vi "Function Generator.vi"() -> ()   [LabVIEW 2024]
uses:
  <vilib>/Instr/_visa.llb/VISA Configure Serial Port (Instr).vi
  <vilib>/measure/NI_MABase.lvlib
panel:
  in  "Tab Control":enum32{"Page 1", "Page 2"}(tab)
  in  "VISA resource name":refnum<visa-resource-name>
  in  "frequency * 100":dbl(knob) scale=0.0..20.0
  in  "signal type":T1(ring)
  in  "stop":bool
  out "Waveform Chart":waveform(dbl)(graph)
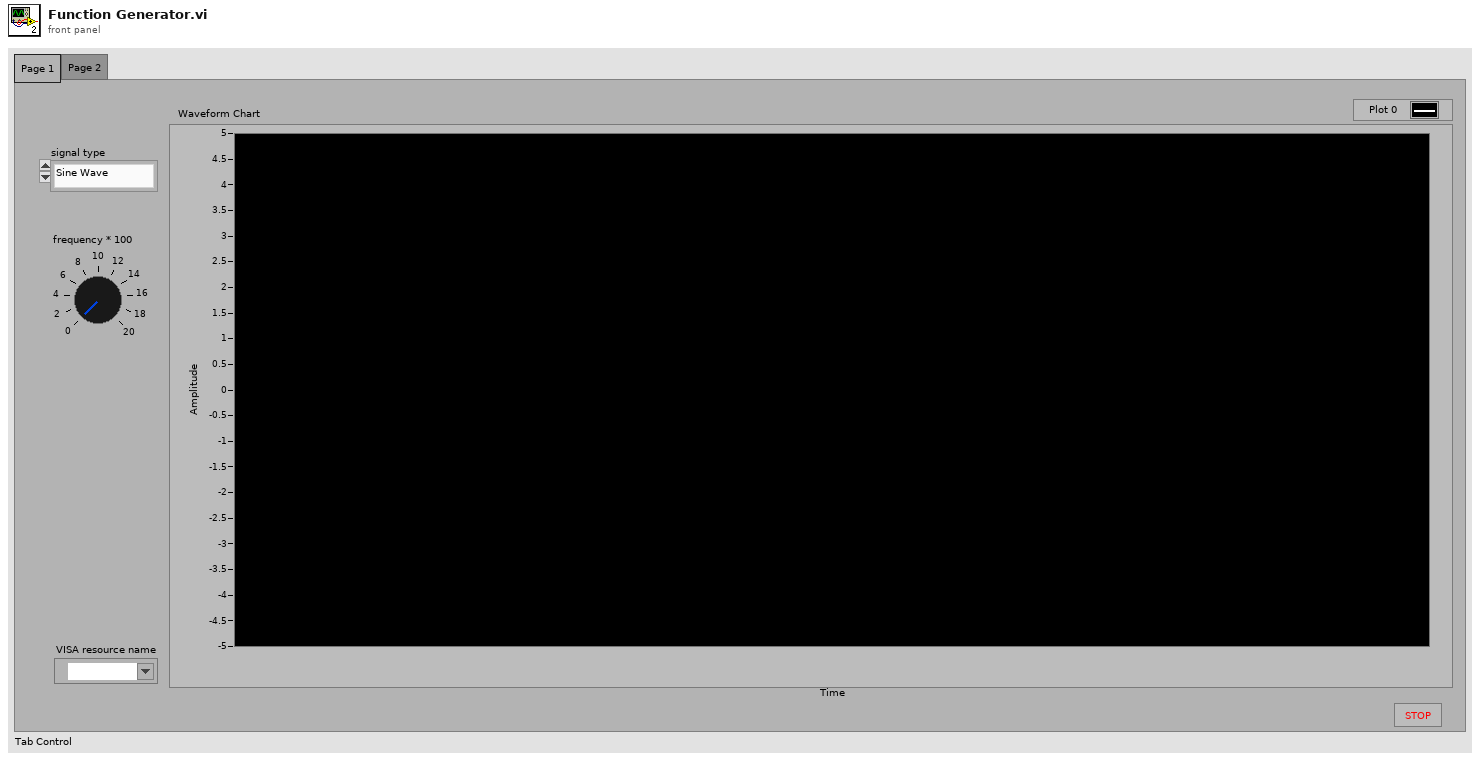
[diagram p1: front panel]
types:
  T1 = enum16{"Sine Wave", "Triangle Wave", "Square Wave", "Sawtooth Wave"}
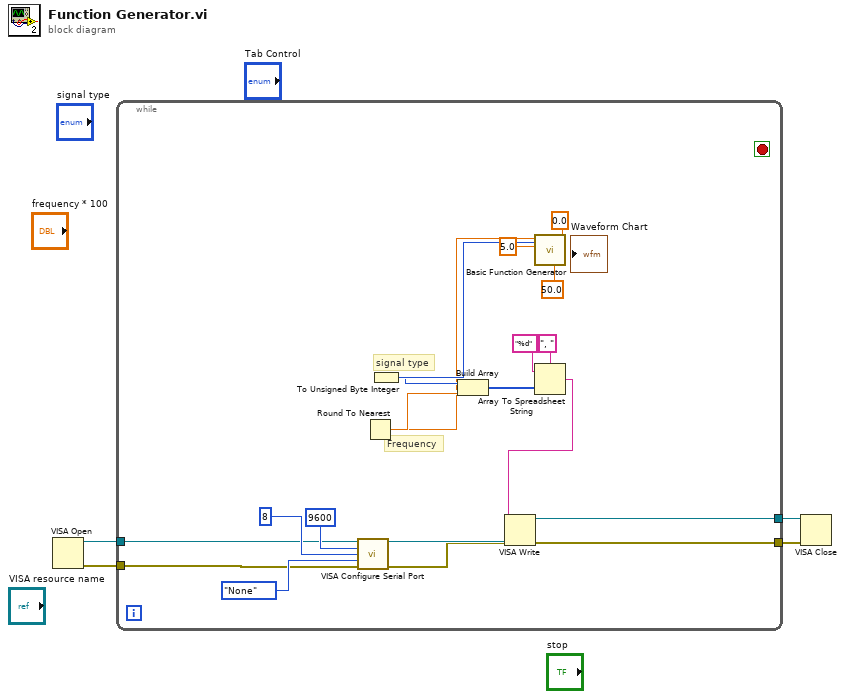
[diagram p0: block diagram]
diagram:
  n1 = VISA Open() -> (VISA resource name=w2:refnum<visa-resource-name>, error out=w1:errorcluster)  [unwired: 5 in]
  n2 = while {
    tunnel: [w24] -> w4
    tunnel: [w23] -> w3
    tunnel: w2 -> [w6]
    tunnel: w1 -> [w5]
    stop <- _ stop-if-true
    # "Frequency"
    # "signal type"
    n3 = call-poly "VISA Configure Serial Port"("VISA resource name"=w6, "baud rate (9600)"=u32 9600, "data bits (8)"=u16 8, "parity (0:none)"=enum16{"None", "Odd", "Even", "Mark", "Space"}."None", "error in (no error)"=w5) -> ("VISA resource name out"=w12:refnum<visa-resource-name>, "error out"=w11:errorcluster)  [unwired: 9 in]
    n4 = call <vilib>:"Basic Function Generator.vi"("offset"=0.0, "square wave duty cycle (%)"=50.0, "amplitude"=5.0) -> ("signal out"=w25:waveform(dbl), "signal type"=w22:T1, "frequency"=w7:dbl)  [unwired: 4 in, 2 out]
    n5 = Round To Nearest(number=w7) -> (nearest integer value=w20:dbl)
    n6 = To Unsigned Byte Integer(number=w22) -> (unsigned 8bit integer=w21:u8)
    n7 = Build Array(w21, w20) -> (w19:u8[])
    n8 = Array To Spreadsheet String(delimiter (Tab)=", ", array=w19, 3:"%d" ("format string")) -> (spreadsheet string=w18:string)
    n9 = VISA Write(VISA resource name=w12, write buffer=w18, error in (no error)=w11) -> (VISA resource name out=w24:refnum<visa-resource-name>, error out=w23:errorcluster)  [unwired: 1 out]
  }
  n10 = VISA Close(VISA resource name=w4, error in (no error)=w3) -> ()  [unwired: 1 out]
